vi "intentoHisto.vi"() -> ()   [LabVIEW 2020]
uses:
  <vilib>/ptbypt/NI_PtbyPt.lvlib
panel:
  out "x+1":i32
  in  "stop":bool
  in  "initialize":bool
  in  "sample length":i32=100
  in  "x":dbl format="%0.2f"
  out "Histogram Graph":T1(graph)
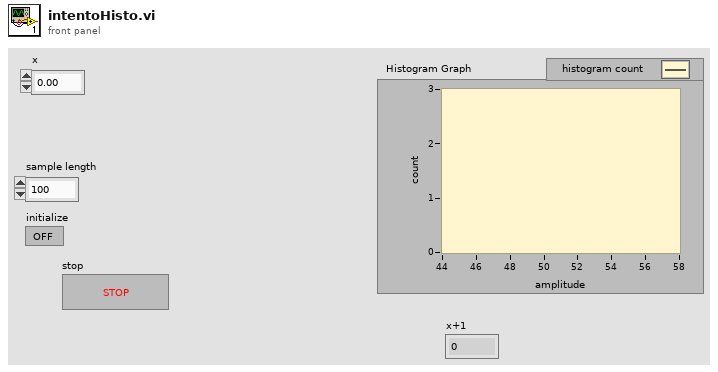
[diagram p1: front panel]
types:
  T1 = cluster{"X Values":dbl[], "Histogram: h(x)":i32[]}
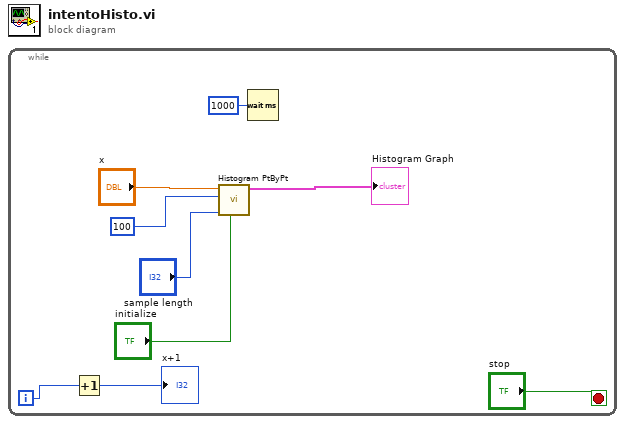
[diagram p0: block diagram]
diagram:
  n1 = while {
    i -> [w2]
    stop <- "stop" stop-if-true
    n2 = Increment(x=w2) -> (x+1=→"x+1":i32)
    n3 = call <vilib>:"Histogram PtByPt.vi"("initialize"="initialize", "sample length"="sample length", "intervals"=100, "x"="x") -> ("Histogram Graph"=→"Histogram Graph":T1)  [unwired: 4 in, 3 out]
    n4 = Wait (ms)(milliseconds to wait=u32 1000) -> ()  [unwired: 1 out]
  }
